vi "FPGA Main.vi"   [LabVIEW 2019]
uses:
  <vilib>/rvi/Emulation/niFpgaGetClockAttributes.vi
  <vilib>/rvi/Emulation/niFpgaSctlEmulationGetInTimedLoop.vi
  <vilib>/rvi/Emulation/niFpgaEmulationReportErrorSimple.vi
  <vilib>/rvi/eio/common/nirviEmuTemplateMethod_errors.vi
  <vilib>/rvi/Emulation/niFpgaCriticalErrorInLSC.vi
  <vilib>/eio/EIONode/EIONode.xnode
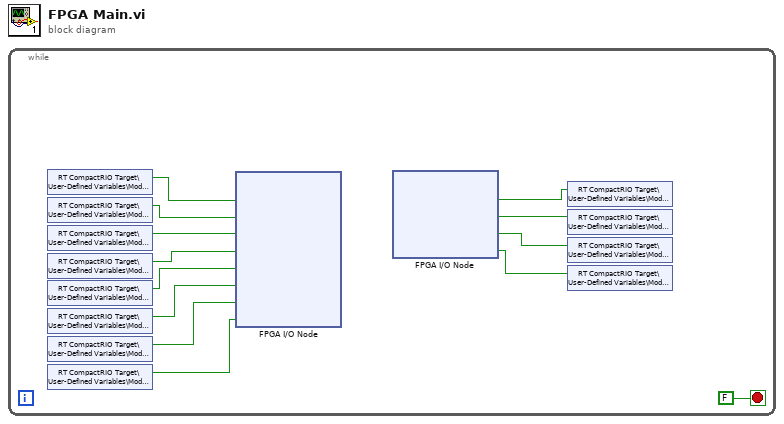
[diagram p0: block diagram]
diagram:
  n1 = while {
    stop <- FALSE stop-if-true
    n2 = shared-variable "RT CompactRIO Target\\User-Defined Variables\\Mod7 DIO0"() -> (w6:bool)  [unwired: 1 in, 1 out]
    n3 = shared-variable "RT CompactRIO Target\\User-Defined Variables\\Mod7 DIO1"() -> (w7:bool)  [unwired: 1 in, 1 out]
    n4 = shared-variable "RT CompactRIO Target\\User-Defined Variables\\Mod7 DIO2"() -> (w8:bool)  [unwired: 1 in, 1 out]
    n5 = shared-variable "RT CompactRIO Target\\User-Defined Variables\\Mod7 DIO3"() -> (w9:bool)  [unwired: 1 in, 1 out]
    n6 = shared-variable "RT CompactRIO Target\\User-Defined Variables\\Mod7 DIO4"() -> (w4:bool)  [unwired: 1 in, 1 out]
    n7 = shared-variable "RT CompactRIO Target\\User-Defined Variables\\Mod7 DIO5"() -> (w3:bool)  [unwired: 1 in, 1 out]
    n8 = shared-variable "RT CompactRIO Target\\User-Defined Variables\\Mod7 DIO6"() -> (w2:bool)  [unwired: 1 in, 1 out]
    n9 = shared-variable "RT CompactRIO Target\\User-Defined Variables\\Mod7 DIO7"() -> (w1:bool)  [unwired: 1 in, 1 out]
    n10 = xnode "FPGA I/O Node"("Mod7/DIO0"=w6, "Mod7/DIO1"=w7, "Mod7/DIO2"=w8, "Mod7/DIO3"=w9, "Mod7/DIO4"=w4, "Mod7/DIO5"=w3, "Mod7/DIO6"=w2, "Mod7/DIO7"=w1) -> ()  [unwired: 8 in, 8 out]
    n11 = xnode "FPGA I/O Node"() -> ("Mod6/DIO0"=w13:bool, "Mod6/DIO1"=w12:bool, "Mod6/DIO2"=w11:bool, "Mod6/DIO3"=w10:bool)  [unwired: 4 in, 4 out]
    n12 = shared-variable "RT CompactRIO Target\\User-Defined Variables\\Mod6 DIO0"(w13) -> ()  [unwired: 1 in, 1 out]
    n13 = shared-variable "RT CompactRIO Target\\User-Defined Variables\\Mod6 DIO1"(w12) -> ()  [unwired: 1 in, 1 out]
    n14 = shared-variable "RT CompactRIO Target\\User-Defined Variables\\Mod6 DIO2"(w11) -> ()  [unwired: 1 in, 1 out]
    n15 = shared-variable "RT CompactRIO Target\\User-Defined Variables\\Mod6 DIO3"(w10) -> ()  [unwired: 1 in, 1 out]
  }
